vi "save roi position.vi"(10 "Gest":string, 11 "input cluster":T1) -> (0 "error out":errorcluster)   [LabVIEW 2022 SP3]
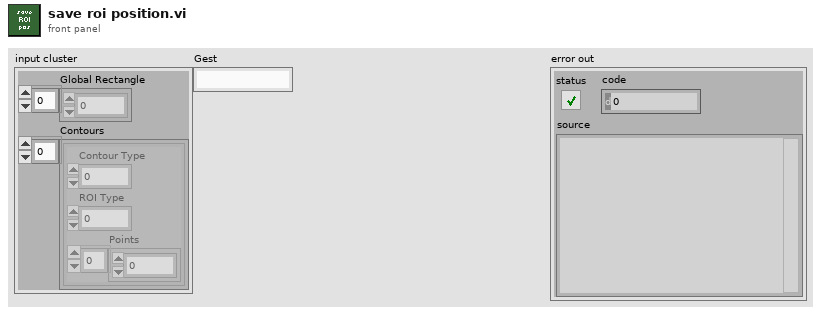
[diagram p1: front panel]
types:
  T1 = cluster{"Global Rectangle":i32[], "Contours":cluster{"Contour Type":u32, "ROI Type":u32, "Points":i32[]}[]}
  T2 = enum16{"open", "replace", "create", "open or create", "replace or create", "replace or create with confirmation"}
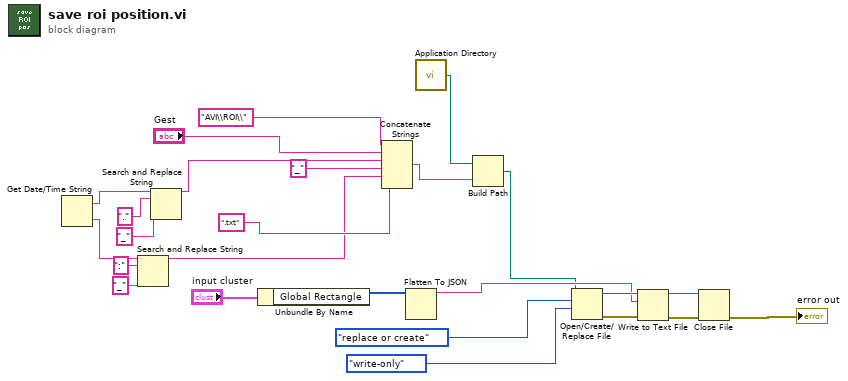
[diagram p0: block diagram]
diagram:
  n1 = Get Date/Time String() -> (date string=w10:string, time string=w4:string)  [unwired: 3 in]
  n2 = Search and Replace String(input string=w4, search string=":", replace string="_" ("replace string (\"\")")) -> (result string=w1:string)  [unwired: 5 in, 3 out]
  n3 = Search and Replace String(input string=w10, search string=".", replace string="_" ("replace string (\"\")")) -> (result string=w9:string)  [unwired: 5 in, 3 out]
  n4 = Unbundle By Name("input cluster") -> ("Global Rectangle"=w25:i32[])
  n5 = Concatenate Strings("AVI\\ROI\\", "Gest", w9, "_" ("string"), w1, ".txt" ("string")) -> (w13:string)
  n6 = Flatten To JSON(anything=w25) -> (JSON string=w21:string)  [unwired: 2 in, 1 out]
  n7 = call <vilib>:"Application Directory.vi"() -> ("Application Directory"=w14:path)
  n8 = Build Path(base path=w14, name or relative path=w13) -> (appended path=w12:path)
  n9 = Open/Create/Replace File(file path (use dialog)=w12, operation (0:open)=T2."replace or create", access (0:read/write)=enum16{"read/write", "read-only", "write-only"}."write-only") -> (refnum out=w22:refnum<file>, error out=w20:errorcluster)  [unwired: 3 in, 1 out]
  n10 = Write to Text File(file (use dialog)=w22, text=w21, error in=w20) -> (refnum out=w19:refnum<file>, error out=w18:errorcluster)  [unwired: 1 in, 1 out]
  n11 = Close File(refnum=w19, error in=w18) -> (error out=→"error out":errorcluster)  [unwired: 1 out]
